vi "FTW-CodeGen-Compare.vi"(0 "State In":T2, 5 "XRef":refnum<vi>, 7 "Data In":T2, 9 "XRefOther":refnum<vi>) -> (4 "Diffs":T1(array[cluster]))   [LabVIEW 2015, in "FTW-dotNet-MySQL-Fetch.xnode"]
uses:
  FTW-dotNet-MySQL-Fetch.xnode
  FTW-CodeGen-State.ctl
panel:
  # "Inputs"
  # "Outputs"
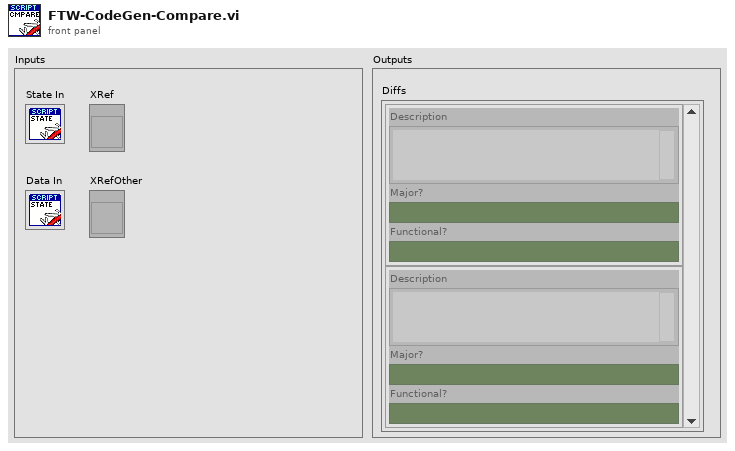
[diagram p1: front panel]
types:
  T1 = cluster{"Description":string, "Major?":bool, "Functional?":bool}[]
  T2 = typedef "FTW-dotNet-MySQL-Fetch.xnode/FTW-CodeGen-State.ctl" = cluster{"Dummy":string}
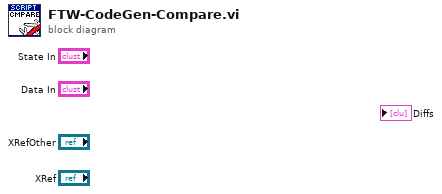
[diagram p0: block diagram]
diagram:
